vi "Close_Interface_Global.vi"(0 "Error In":errorcluster caption="Fehler (Eingang, kein Fehler)") -> ()   [LabVIEW 2016]
uses:
  Utility/Global_Sensor.vi
  Utility/Global Constants.vi
  Program Files/MicroEpsilon/MEDAQLib-3.2.3.19901/Samples/LabView/MEDAQLib/MEDAQLib.lvlib
panel:
  out "Close Errors":string
  out "Release Errors":string
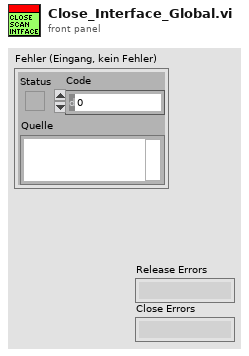
[diagram p1: front panel]
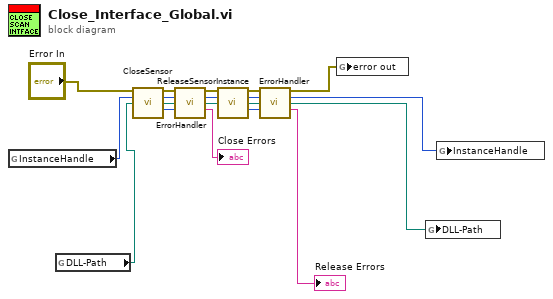
[diagram p0: block diagram]
diagram:
  n1 = global read "Global_Sensor.vi" "InstanceHandle"() -> (w5:u32)
  n2 = global read "Global_Sensor.vi" "DLL-Path"() -> (w4:path)
  n3 = call "CloseSensor.vi"("Fehler (Eingang, kein Fehler)"="Error In", "instanceHandle"=w5, "DLL-Path"=w4) -> ("Fehler (Ausgang)"=w19:errorcluster, "instanceHandle"=w18:u32, "DLL-Path"=w17:path, "ERR_CODE"=w16:i32)  [unwired: 9 in]
  n4 = call "ErrorHandler.vi"("Fehler (Eingang, kein Fehler)"=w19, "instanceHandle"=w18, "DLL-Path"=w17, "ERR_CODE"=w16) -> ("Fehler (Ausgang)"=w15:errorcluster, "instanceHandle"=w14:u32, "DLL-Path"=w13:path, "errText"=→"Close Errors":string)  [unwired: 8 in]
  n5 = call "ReleaseSensorInstance.vi"("Fehler (Eingang, kein Fehler)"=w15, "instanceHandle"=w14, "DLL-Path"=w13) -> ("Fehler (Ausgang)"=w12:errorcluster, "instanceHandle"=w11:u32, "DLL-Path"=w10:path, "ERR_CODE"=w9:i32)  [unwired: 9 in]
  n6 = call "ErrorHandler.vi"("Fehler (Eingang, kein Fehler)"=w12, "instanceHandle"=w11, "DLL-Path"=w10, "ERR_CODE"=w9) -> ("Fehler (Ausgang)"=w6:errorcluster, "instanceHandle"=w3:u32, "DLL-Path"=w2:path, "errText"=→"Release Errors":string)  [unwired: 8 in]
  n7 = global write "Global Constants.vi" "error out"(w6) -> ()
  n8 = global write "Global_Sensor.vi" "DLL-Path"(w2) -> ()
  n9 = global write "Global_Sensor.vi" "InstanceHandle"(w3) -> ()
